vi "Controller Tuning.vi"() -> ()   [LabVIEW 2015]
doc: "Simple controller tuning VI."
uses:
  PL Bronkhorst ProPar.lvclass
panel:
  in  "control mode":u8(ring) items=["setpoint"=0, "close valve"=3, "controller idle"=4, "purge valve"=8, "valve stearing"=20]
  in  "setpoint ramp time, s":sgl
  in  "valve opening offset":sgl
  out "chart":T1(graph)
  in  "valve, %":sgl
  in  "controller response":cluster{"open":u8, "normal":u8, "stable":u8}
  in  "PID":cluster{"Kp":sgl, "Ti":sgl, "Td":sgl}
  out "fluid name":string
  in  "wink":bool
  in  "setpoint, %":sgl
  out "measured value, %":sgl
  out "user tag":string
  out "id string":string
  in  "node":u8
  out "ProPar":refnum<class "PL Bronkhorst ProPar.lvclass">
  in  "baud rate":u32=38400
  in  "port":refnum<visa-resource-name>
  out "error":errorcluster
  in  "stop":bool
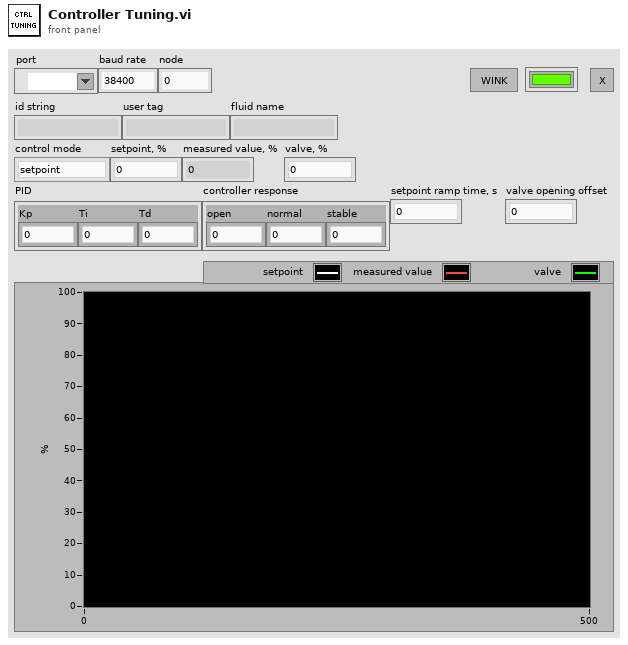
[diagram p1: front panel]
types:
  T1 = cluster{"setpoint":sgl, "measured value":sgl, "valve position, %":sgl}
  T2 = cluster{"setpoint":sgl, "measured value":sgl, "valve position, %":sgl}[]
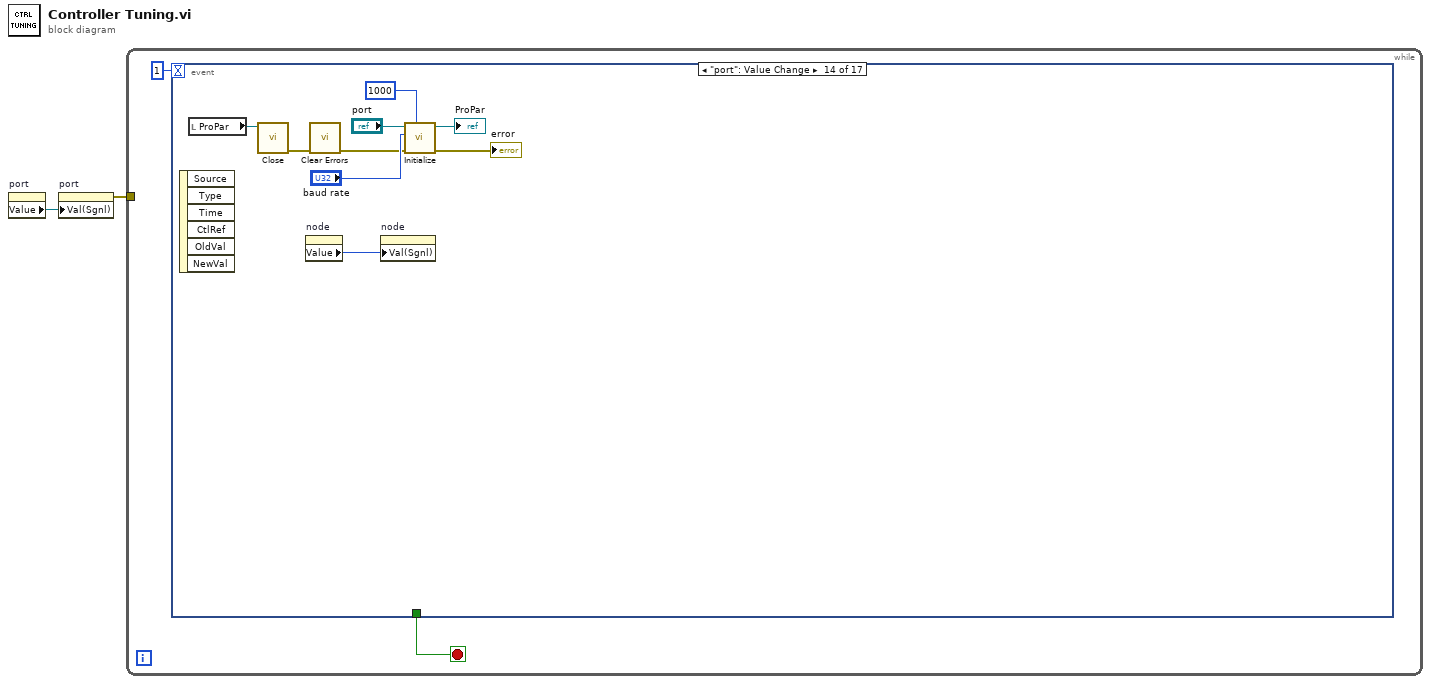
[diagram p0: block diagram]
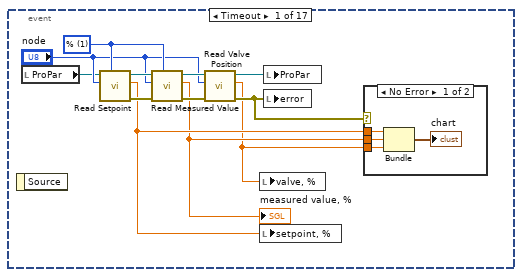
[diagram p2: hidden frame]
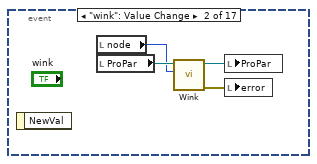
[diagram p4: hidden frame]
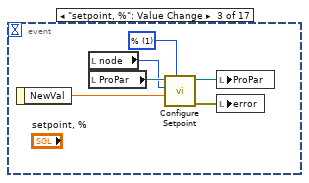
[diagram p5: hidden frame]
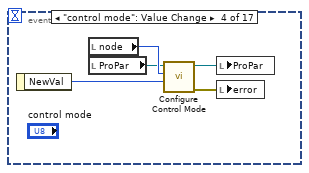
[diagram p6: hidden frame]
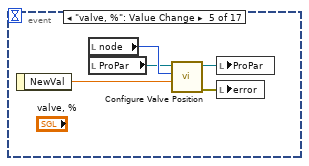
[diagram p7: hidden frame]
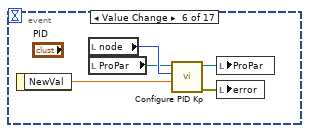
[diagram p8: hidden frame]
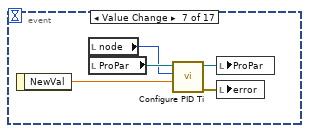
[diagram p9: hidden frame]
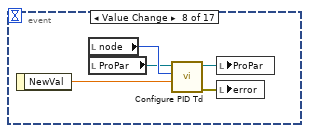
[diagram p10: hidden frame]
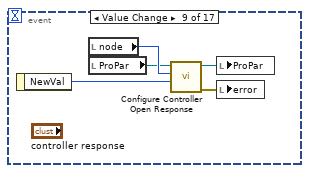
[diagram p11: hidden frame]
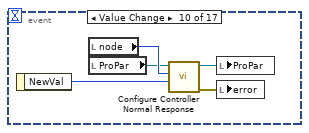
[diagram p12: hidden frame]
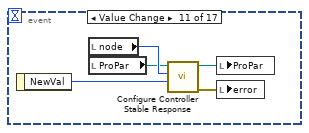
[diagram p13: hidden frame]
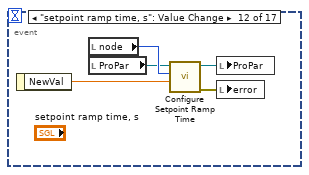
[diagram p14: hidden frame]
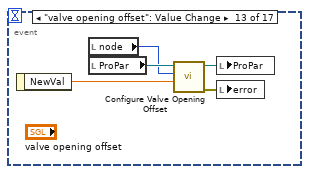
[diagram p15: hidden frame]
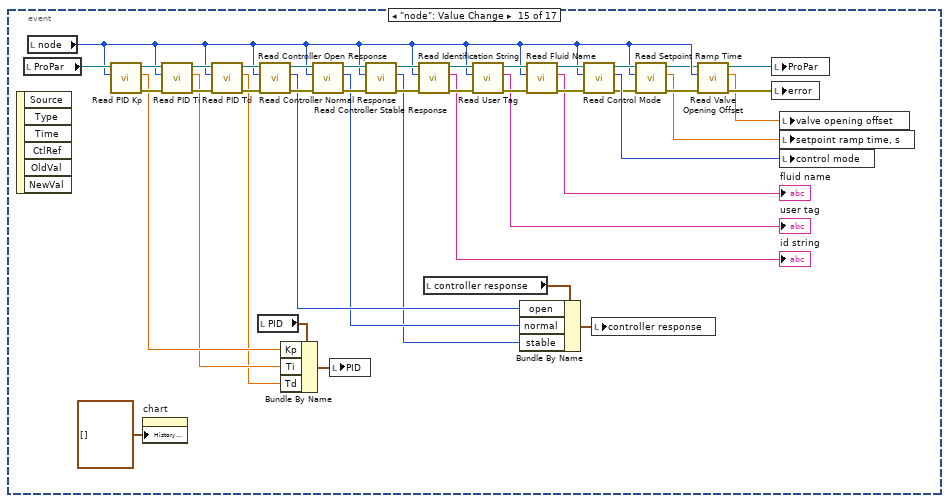
[diagram p16: hidden frame]
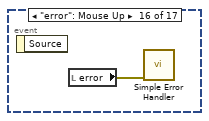
[diagram p17: hidden frame]
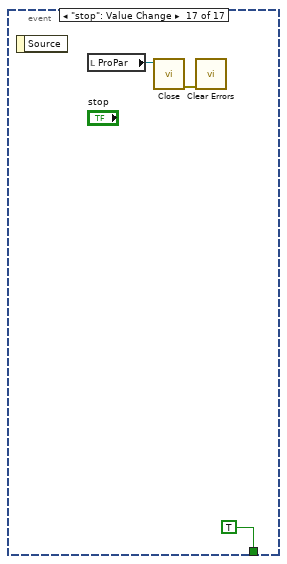
[diagram p18: hidden frame]
diagram:
  n1 = property on="port" class="VISAName"() -> ("Value"=w1:refnum<visa-resource-name>)  [unwired: 2 in, 2 out]
  n2 = property on="port" class="VISAName"("Val(Sgnl)"=w1) -> (error out=w2:errorcluster)  [unwired: 2 in, 1 out]
  n3 = while {
    tunnel: w2 -> [_]
    stop <- w3 stop-if-true
    n4 = event shown="[13] \"port\": Value Change" {
      selector: _ -> [_ _ _ _ _ _ _ _ _ _ _ _ _ _ _ _ _]
      dyn-events: _ -> [_ _ _ _ _ _ _ _ _ _ _ _ _ _ _ _ _]
      timeout: 1 -> [_ _ _ _ _ _ _ _ _ _ _ _ _ _ _ _ _]
      tunnel: [_ _ _ _ _ _ _ _ _ _ _ _ _ _ _ _ TRUE ("stop")] -> w3
      event Timeout {
        w14 = u16 1 items=["capacity unit", "%"] ("unit (capacity unit)")
        n5 = event-data() -> ()  [unwired: 1 in, 1 out]
        n6 = local read "ProPar"() -> (w10:refnum<class "PL Bronkhorst ProPar.lvclass">)
        n7 = call "Read Setpoint.vi"("unit (capacity unit)"=w14, "node"="node", "ProPar in"=w10) -> ("error out"=w16:errorcluster, "setpoint"=w7:sgl, "ProPar out"=w15:refnum<class "PL Bronkhorst ProPar.lvclass">)  [unwired: 6 in]
        n8 = call "Read Measured Value.vi"("unit (capacity unit)"=w14, "error in (no error)"=w16, "node"="node", "ProPar in"=w15) -> ("error out"=w12:errorcluster, "measured value"=w6:sgl, "ProPar out"=w13:refnum<class "PL Bronkhorst ProPar.lvclass">)  [unwired: 5 in]
        "measured value, %" <- w6
        n9 = call "Read Valve Position.vi"("error in (no error)"=w12, "node"="node", "ProPar in"=w13) -> ("error out"=w8:errorcluster, "valve position, %"=w5:sgl, "ProPar out"=w9:refnum<class "PL Bronkhorst ProPar.lvclass">)  [unwired: 6 in]
        n10 = local write "valve, %"(w5) -> ()
        n11 = local write "setpoint, %"(w7) -> ()
        n12 = local write "ProPar"(w9) -> ()
        n13 = local write "error"(w8) -> ()
        n14 = case shown="No Error" w8 {
          tunnel: w7 -> [w20 _]
          tunnel: w6 -> [w19 _]
          tunnel: w5 -> [w18 _]
          frame No Error {
            n15 = Bundle("setpoint"=w20, "measured value"=w19, "valve position, %"=w18) -> (→"chart":T1)  [unwired: 1 in]
          }
          frame Error {
          }
        }
      }
      event "wink": Value Change {
        n16 = event-data() -> ()  [unwired: 1 in, 1 out]
        n17 = local read "node"() -> (w21:u8)
        n18 = local read "ProPar"() -> (w22:refnum<class "PL Bronkhorst ProPar.lvclass">)
        n19 = call "Wink.vi"("node"=w21, "ProPar in"=w22) -> ("error out"=w23:errorcluster, "ProPar out"=w24:refnum<class "PL Bronkhorst ProPar.lvclass">)  [unwired: 8 in]
        n20 = local write "ProPar"(w24) -> ()
        n21 = local write "error"(w23) -> ()
      }
      event "setpoint, %": Value Change {
        w25 = u16 1 items=["capacity unit", "%"] ("unit (capacity unit)")
        n22 = event-data() -> ("NewVal"=w28:sgl)  [unwired: 1 in]
        n23 = local read "node"() -> (w26:u8)
        n24 = local read "ProPar"() -> (w27:refnum<class "PL Bronkhorst ProPar.lvclass">)
        n25 = call "Configure Setpoint.vi"("unit (capacity unit)"=w25, "setpoint"=w28, "node"=w26, "ProPar in"=w27) -> ("error out"=w29:errorcluster, "ProPar out"=w30:refnum<class "PL Bronkhorst ProPar.lvclass">)  [unwired: 6 in]
        n26 = local write "ProPar"(w30) -> ()
        n27 = local write "error"(w29) -> ()
      }
      event "control mode": Value Change {
        n28 = event-data() -> ("NewVal"=w33:u8)  [unwired: 1 in]
        n29 = local read "node"() -> (w32:u8)
        n30 = local read "ProPar"() -> (w31:refnum<class "PL Bronkhorst ProPar.lvclass">)
        n31 = call "Configure Control Mode.vi"("control mode"=w33, "node"=w32, "ProPar in"=w31) -> ("error out"=w34:errorcluster, "ProPar out"=w35:refnum<class "PL Bronkhorst ProPar.lvclass">)  [unwired: 7 in]
        n32 = local write "ProPar"(w35) -> ()
        n33 = local write "error"(w34) -> ()
      }
      event "valve, %": Value Change {
        n34 = event-data() -> ("NewVal"=w39:sgl)  [unwired: 1 in]
        n35 = local read "node"() -> (w37:u8)
        n36 = local read "ProPar"() -> (w36:refnum<class "PL Bronkhorst ProPar.lvclass">)
        n37 = call "Configure Valve Position.vi"("valve position, %"=w39, "node"=w37, "ProPar in"=w36) -> ("error out"=w38:errorcluster, "ProPar out"=w40:refnum<class "PL Bronkhorst ProPar.lvclass">)  [unwired: 7 in]
        n38 = local write "ProPar"(w40) -> ()
        n39 = local write "error"(w38) -> ()
      }
      event "PID.Kp": Value Change {
        n40 = event-data() -> ("NewVal"=w43:sgl)  [unwired: 1 in]
        n41 = local read "node"() -> (w42:u8)
        n42 = local read "ProPar"() -> (w41:refnum<class "PL Bronkhorst ProPar.lvclass">)
        n43 = call "Configure PID Kp.vi"("PID Kp"=w43, "node"=w42, "ProPar in"=w41) -> ("error out"=w44:errorcluster, "ProPar out"=w45:refnum<class "PL Bronkhorst ProPar.lvclass">)  [unwired: 7 in]
        n44 = local write "ProPar"(w45) -> ()
        n45 = local write "error"(w44) -> ()
      }
      event "PID.Ti": Value Change {
        n46 = event-data() -> ("NewVal"=w47:sgl)  [unwired: 1 in]
        n47 = local read "node"() -> (w46:u8)
        n48 = local read "ProPar"() -> (w50:refnum<class "PL Bronkhorst ProPar.lvclass">)
        n49 = call "Configure PID Ti.vi"("PID Ti, s"=w47, "node"=w46, "ProPar in"=w50) -> ("error out"=w48:errorcluster, "ProPar out"=w49:refnum<class "PL Bronkhorst ProPar.lvclass">)  [unwired: 7 in]
        n50 = local write "ProPar"(w49) -> ()
        n51 = local write "error"(w48) -> ()
      }
      event "PID.Td": Value Change {
        n52 = event-data() -> ("NewVal"=w53:sgl)  [unwired: 1 in]
        n53 = local read "node"() -> (w52:u8)
        n54 = local read "ProPar"() -> (w51:refnum<class "PL Bronkhorst ProPar.lvclass">)
        n55 = call "Configure PID Td.vi"("PID Td, s"=w53, "node"=w52, "ProPar in"=w51) -> ("error out"=w54:errorcluster, "ProPar out"=w55:refnum<class "PL Bronkhorst ProPar.lvclass">)  [unwired: 7 in]
        n56 = local write "ProPar"(w55) -> ()
        n57 = local write "error"(w54) -> ()
      }
      event "controller response.open": Value Change {
        n58 = event-data() -> ("NewVal"=w58:u8)  [unwired: 1 in]
        n59 = local read "node"() -> (w57:u8)
        n60 = local read "ProPar"() -> (w56:refnum<class "PL Bronkhorst ProPar.lvclass">)
        n61 = call "Configure Controller Open Response.vi"("open response"=w58, "node"=w57, "ProPar in"=w56) -> ("error out"=w59:errorcluster, "ProPar out"=w60:refnum<class "PL Bronkhorst ProPar.lvclass">)  [unwired: 7 in]
        n62 = local write "ProPar"(w60) -> ()
        n63 = local write "error"(w59) -> ()
      }
      event "controller response.normal": Value Change {
        n64 = event-data() -> ("NewVal"=w63:u8)  [unwired: 1 in]
        n65 = local read "node"() -> (w62:u8)
        n66 = local read "ProPar"() -> (w61:refnum<class "PL Bronkhorst ProPar.lvclass">)
        n67 = call "Configure Controller Normal Response.vi"("normal response"=w63, "node"=w62, "ProPar in"=w61) -> ("error out"=w64:errorcluster, "ProPar out"=w65:refnum<class "PL Bronkhorst ProPar.lvclass">)  [unwired: 7 in]
        n68 = local write "ProPar"(w65) -> ()
        n69 = local write "error"(w64) -> ()
      }
      event "controller response.stable": Value Change {
        n70 = event-data() -> ("NewVal"=w68:u8)  [unwired: 1 in]
        n71 = local read "node"() -> (w67:u8)
        n72 = local read "ProPar"() -> (w66:refnum<class "PL Bronkhorst ProPar.lvclass">)
        n73 = call "Configure Controller Stable Response.vi"("stable response"=w68, "node"=w67, "ProPar in"=w66) -> ("error out"=w69:errorcluster, "ProPar out"=w70:refnum<class "PL Bronkhorst ProPar.lvclass">)  [unwired: 7 in]
        n74 = local write "ProPar"(w70) -> ()
        n75 = local write "error"(w69) -> ()
      }
      event "setpoint ramp time, s": Value Change {
        n76 = event-data() -> ("NewVal"=w73:sgl)  [unwired: 1 in]
        n77 = local read "node"() -> (w72:u8)
        n78 = local read "ProPar"() -> (w71:refnum<class "PL Bronkhorst ProPar.lvclass">)
        n79 = call "Configure Setpoint Ramp Time.vi"("setpoint ramp time, s"=w73, "node"=w72, "ProPar in"=w71) -> ("error out"=w74:errorcluster, "ProPar out"=w75:refnum<class "PL Bronkhorst ProPar.lvclass">)  [unwired: 7 in]
        n80 = local write "ProPar"(w75) -> ()
        n81 = local write "error"(w74) -> ()
      }
      event "valve opening offset": Value Change {
        n82 = event-data() -> ("NewVal"=w77:sgl)  [unwired: 1 in]
        n83 = local read "node"() -> (w76:u8)
        n84 = local read "ProPar"() -> (w80:refnum<class "PL Bronkhorst ProPar.lvclass">)
        n85 = call "Configure Valve Opening Offset.vi"("offset"=w77, "node"=w76, "ProPar in"=w80) -> ("error out"=w78:errorcluster, "ProPar out"=w79:refnum<class "PL Bronkhorst ProPar.lvclass">)  [unwired: 7 in]
        n86 = local write "ProPar"(w79) -> ()
        n87 = local write "error"(w78) -> ()
      }
      event "port": Value Change {
        n88 = event-data() -> ()  [unwired: 1 in, 6 out]
        n89 = local read "ProPar"() -> (w84:refnum<class "PL Bronkhorst ProPar.lvclass">)
        n90 = call "Close.vi"("ProPar in"=w84) -> ("error out"=w86:errorcluster)  [unwired: 10 in]
        n91 = property on="node" class="DigNum (strict)"() -> ("Value"=w81:u8)  [unwired: 2 in, 2 out]
        n92 = call <vilib>:"Clear Errors.vi"("error in (no error)"=w86) -> ("error out"=w83:errorcluster)  [unwired: 5 in, 1 out]
        n93 = property on="node" class="DigNum (strict)"("Val(Sgnl)"=w81) -> ()  [unwired: 2 in, 2 out]
        n94 = call "Initialize.vi"("timeout, ms (1000)"=u32 1000, "error in (no error)"=w83, "baud rate (38400)"="baud rate", "port"="port") -> ("error out"=→"error":errorcluster, "ProPar out"=→"ProPar":refnum<class "PL Bronkhorst ProPar.lvclass">)  [unwired: 6 in]
      }
      event "node": Value Change {
        n95 = event-data() -> ()  [unwired: 1 in, 6 out]
        n96 = local read "ProPar"() -> (w116:refnum<class "PL Bronkhorst ProPar.lvclass">)
        n97 = local read "node"() -> (w97:u8)
        n98 = call "Read PID Kp.vi"("node"=w97, "ProPar in"=w116) -> ("error out"=w127:errorcluster, "PID Kp"=w125:sgl, "ProPar out"=w128:refnum<class "PL Bronkhorst ProPar.lvclass">)  [unwired: 7 in]
        n99 = property on="chart" class="WFChart (strict)"("History Data"=T2 []) -> ()  [unwired: 2 in, 2 out]
        n100 = call "Read PID Ti.vi"("error in (no error)"=w127, "node"=w97, "ProPar in"=w128) -> ("error out"=w126:errorcluster, "PID Ti"=w112:sgl, "ProPar out"=w129:refnum<class "PL Bronkhorst ProPar.lvclass">)  [unwired: 6 in]
        n101 = call "Read PID Td.vi"("error in (no error)"=w126, "node"=w97, "ProPar in"=w129) -> ("error out"=w119:errorcluster, "PID Td"=w111:sgl, "ProPar out"=w124:refnum<class "PL Bronkhorst ProPar.lvclass">)  [unwired: 6 in]
        n102 = local read "PID"() -> (w110:cluster{"Kp":sgl, "Ti":sgl, "Td":sgl})
        n103 = call "Read Controller Open Response.vi"("error in (no error)"=w119, "node"=w97, "ProPar in"=w124) -> ("error out"=w120:errorcluster, "open response"=w108:u8, "ProPar out"=w123:refnum<class "PL Bronkhorst ProPar.lvclass">)  [unwired: 6 in]
        n104 = Bundle By Name(cluster=w110, "Kp"=w125, "Ti"=w112, "Td"=w111) -> (w109:cluster{"Kp":sgl, "Ti":sgl, "Td":sgl})
        n105 = call "Read Controller Normal Response.vi"("error in (no error)"=w120, "node"=w97, "ProPar in"=w123) -> ("error out"=w121:errorcluster, "normal response"=w105:u8, "ProPar out"=w122:refnum<class "PL Bronkhorst ProPar.lvclass">)  [unwired: 6 in]
        n106 = local write "PID"(w109) -> ()
        n107 = call "Read Controller Stable Response.vi"("error in (no error)"=w121, "node"=w97, "ProPar in"=w122) -> ("error out"=w117:errorcluster, "stable response"=w104:u8, "ProPar out"=w118:refnum<class "PL Bronkhorst ProPar.lvclass">)  [unwired: 6 in]
        n108 = call "Read Identification String.vi"("error in (no error)"=w117, "node"=w97, "ProPar in"=w118) -> ("error out"=w132:errorcluster, "id string"=→"id string":string, "ProPar out"=w115:refnum<class "PL Bronkhorst ProPar.lvclass">)  [unwired: 6 in]
        n109 = local read "controller response"() -> (w107:cluster{"open":u8, "normal":u8, "stable":u8})
        n110 = call "Read User Tag.vi"("error in (no error)"=w132, "node"=w97, "ProPar in"=w115) -> ("error out"=w131:errorcluster, "user tag"=→"user tag":string, "ProPar out"=w114:refnum<class "PL Bronkhorst ProPar.lvclass">)  [unwired: 6 in]
        n111 = Bundle By Name(cluster=w107, "open"=w108, "normal"=w105, "stable"=w104) -> (w106:cluster{"open":u8, "normal":u8, "stable":u8})
        n112 = call "Read Fluid Name.vi"("error in (no error)"=w131, "node"=w97, "ProPar in"=w114) -> ("error out"=w130:errorcluster, "fluid name"=→"fluid name":string, "ProPar out"=w113:refnum<class "PL Bronkhorst ProPar.lvclass">)  [unwired: 6 in]
        n113 = call "Read Control Mode.vi"("error in (no error)"=w130, "node"=w97, "ProPar in"=w113) -> ("error out"=w98:errorcluster, "control mode"=w103:u8, "ProPar out"=w99:refnum<class "PL Bronkhorst ProPar.lvclass">)  [unwired: 6 in]
        n114 = local write "controller response"(w106) -> ()
        n115 = call "Read Setpoint Ramp Time.vi"("error in (no error)"=w98, "node"=w97, "ProPar in"=w99) -> ("error out"=w93:errorcluster, "setpoint ramp time, s"=w91:sgl, "ProPar out"=w96:refnum<class "PL Bronkhorst ProPar.lvclass">)  [unwired: 6 in]
        n116 = call "Read Valve Opening Offset.vi"("error in (no error)"=w93, "node"=w97, "ProPar in"=w96) -> ("error out"=w94:errorcluster, "offset"=w92:sgl, "ProPar out"=w95:refnum<class "PL Bronkhorst ProPar.lvclass">)  [unwired: 6 in]
        n117 = local write "ProPar"(w95) -> ()
        n118 = local write "error"(w94) -> ()
        n119 = local write "valve opening offset"(w92) -> ()
        n120 = local write "setpoint ramp time, s"(w91) -> ()
        n121 = local write "control mode"(w103) -> ()
      }
      event "error": Mouse Up {
        n122 = event-data() -> ()  [unwired: 1 in, 1 out]
        n123 = local read "error"() -> (w133:errorcluster)
        n124 = call <vilib>:"Simple Error Handler.vi"("error in (no error)"=w133) -> ()  [unwired: 4 in, 5 out]
      }
      event "stop": Value Change {
        n125 = event-data() -> ()  [unwired: 1 in, 1 out]
        n126 = local read "ProPar"() -> (w135:refnum<class "PL Bronkhorst ProPar.lvclass">)
        n127 = call "Close.vi"("ProPar in"=w135) -> ("error out"=w134:errorcluster)  [unwired: 10 in]
        n128 = call <vilib>:"Clear Errors.vi"("error in (no error)"=w134) -> ()  [unwired: 5 in, 2 out]
      }
    }
  }
